vi "2022SignalManipulation_SINGLECHANNEL.vi"(9 "Cold Junction Temp":dbl, 11 "Data":dbl[][](array[numeric])) -> (3 "Array":dbl[](array[numeric]))   [LabVIEW 2021]
panel:
  out "Array 3":dbl[](array[numeric])
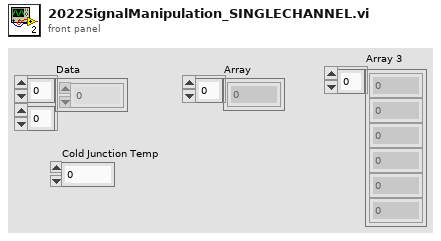
[diagram p1: front panel]
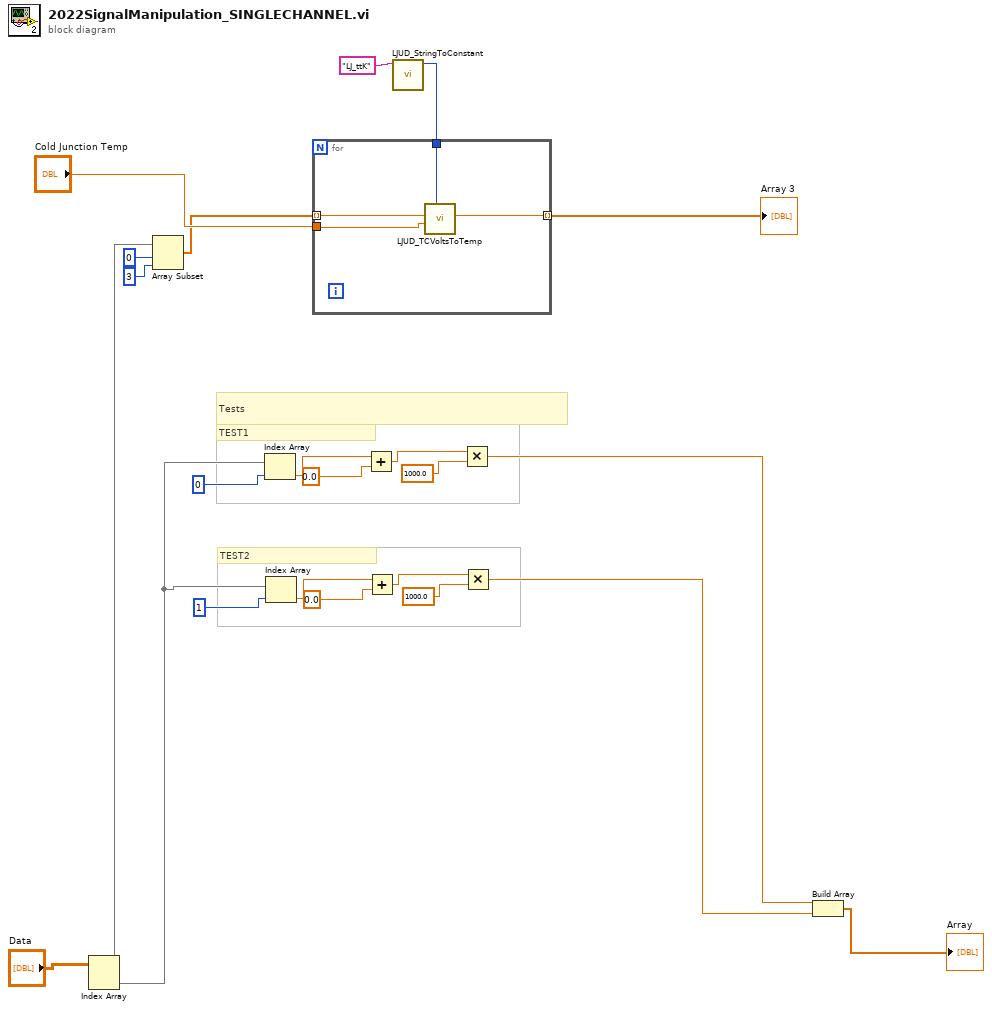
[diagram p0: block diagram]
diagram:
  # "TEST2"
  # "Tests"
  # "TEST1"
  n1 = Index Array(array="Data") -> (element=w2:dbl[])  [unwired: 2 in]
  n2 = Array Subset(array=w2, index=0, length=3) -> (w12:dbl[])
  n3 = Index Array(array=w2, index=0 ("index (col)")) -> (element=w19:dbl)
  n4 = Index Array(array=w2, index=1 ("index (col)")) -> (element=w4:dbl)
  n5 = Add(x=w19, y=0.0) -> (x+y=w22:dbl)
  n6 = Add(x=w4, y=0.0) -> (x+y=w7:dbl)
  n7 = call "LJUD_StringToConstant.vi"("String"="LJ_ttK") -> ("Constant Number"=w10:i32)  [unwired: 9 in, 1 out]
  n8 = for {
    tunnel: "Cold Junction Temp" -> [w25]
    tunnel: w12 -> [w26] mode=indexing
    tunnel: [w23] -> w11 mode=indexing
    tunnel: w10 -> [w24]
    n9 = call "LJUD_TCVoltsToTemp.vi"("TCType"=w24, "CJTempK"=w25, "TCVolts"=w26) -> ("TCTempC"=w23:dbl)  [unwired: 5 in, 3 out]
  }
  "Array 3" <- w11
  n10 = Multiply(x=w22, y=1000.0) -> (x*y=w9:dbl)
  n11 = Multiply(x=w7, y=1000.0) -> (x*y=w1:dbl)
  n12 = Build Array(w9, w1) -> (→"Array":dbl[])
